vi "DialogCreateClass_FilterAndOrderClassTemplates.vi"(8 "error in (no error)":errorcluster, 11 "AllTemplatesForThisProvider/InheritanceType(Base/Sub)":T1[](array[typedef])) -> (0 "error out":errorcluster, 2 "NewOrderIndex":i32[](array[numeric]), 3 "FilteredTemplates":T1[](array[typedef]))   [LabVIEW 2020, in "ClassWriterNative.lvclass"]
uses:
  <resource>/Framework/Providers/Open_GDS/ClassProviders/Provider_LvNativeClass/ClassWriterNative_class/ClassWriterNative.lvclass
  <resource>/Framework/Providers/Open_GDS/ClassProviders/Provider_BaseClassInterface/ClassTemplateType.ctl
  <resource>/Framework/Providers/Open_GDS/ClassProviders/Provider_BaseClassInterface/ClassWriter_class/ClassWriter.lvclass
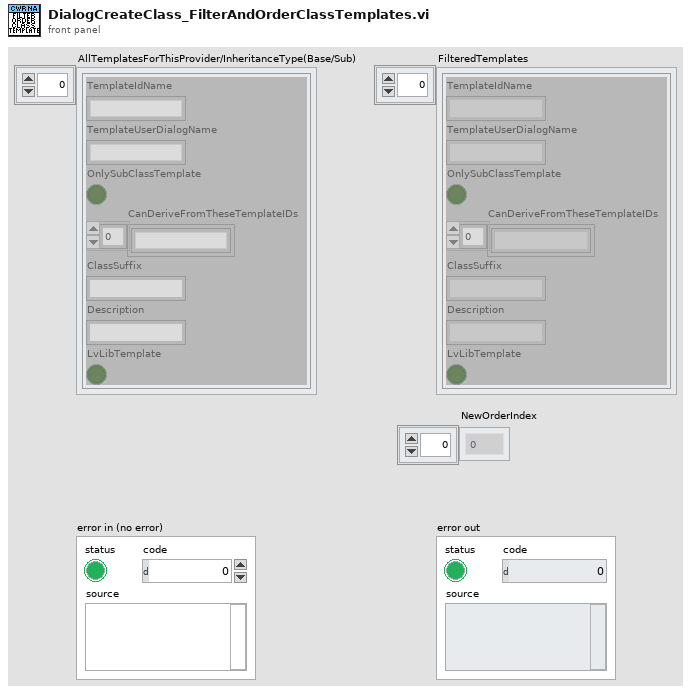
[diagram p1: front panel]
types:
  T1 = typedef "ClassWriter.lvclass/ClassTemplateType.ctl" = cluster{"TemplateIdName":string, "TemplateUserDialogName":string, "OnlySubClassTemplate":bool, "CanDeriveFromTheseTemplateIDs":string[], "ClassSuffix":string, "Description":string, "LvLibTemplate":bool}
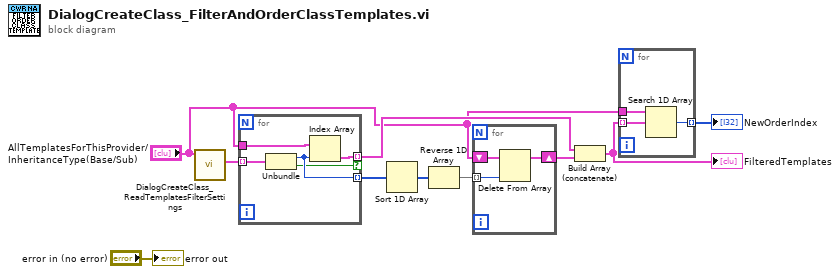
[diagram p0: block diagram]
diagram:
  n1 = call <resource>:"DialogCreateClass_ReadTemplatesFilterSettings.vi"("AllTemplatesForThisProvider/InheritanceType(Base/Sub)"="AllTemplatesForThisProvider/InheritanceType(Base/Sub)") -> ("FilterSettings(OrderIndex,Active)"=w9:cluster{"Numeric":i32, "Checkbox":bool}[])  [unwired: 9 in, 1 out]
  n2 = for {
    tunnel: w9 -> [w15] mode=indexing
    tunnel: "AllTemplatesForThisProvider/InheritanceType(Base/Sub)" -> [w14]
    tunnel: [w11] -> w5 mode=indexing if=w12
    tunnel: [w13] -> w6 mode=indexing
    n3 = Unbundle(w15) -> ("Numeric"=w13:i32, "Checkbox"=w12:bool)
    n4 = Index Array(array=w14, index=w13) -> (element=w11:T1)
  }
  n5 = Sort 1D Array(array=w6) -> (sorted array=w7:i32[])
  n6 = Reverse 1D Array(array=w7) -> (reversed array=w8:i32[])
  n7 = for {
    shift-right: [w16] -> w4
    shift-left: "AllTemplatesForThisProvider/InheritanceType(Base/Sub)" -> [w18]
    tunnel: w8 -> [w17] mode=indexing
    n8 = Delete From Array(array=w18, index=w17) -> (array with subset deleted=w16:T1[])  [unwired: 1 in, 1 out]
  }
  n9 = Build Array (concatenate)(w5, w4) -> (w3:T1[])
  "FilteredTemplates" <- w3
  n10 = for {
    tunnel: w3 -> [w21] mode=indexing
    tunnel: "AllTemplatesForThisProvider/InheritanceType(Base/Sub)" -> [w20]
    tunnel: [w19] -> w1 mode=indexing
    n11 = Search 1D Array(1D array=w20, element=w21) -> (index of element=w19:i32)  [unwired: 1 in]
  }
  "NewOrderIndex" <- w1
  "error out" <- "error in (no error)"
